vi "READ FGV.vi"(7 "Enum":T1=enum."WRITE", 8 "error in (no error)":errorcluster) -> (0 "error out":errorcluster, 3 "data":dbl[](array[numeric]) format="%.2f")   [LabVIEW 2025]
uses:
  FGV States.ctl
  CAN Write Data/Application/Common VIs/Read File Data.ctl
  <vilib>/xnet/xnet.llb/XNET Read (Signal Single-point).vi
  <vilib>/xnet/xnet.llb/XNET Create Session (Signal Input Single-point).vi
panel:
  out "DBC FUNCTIONS OUT":string[](array[string])
  out "session out 2":refnum<k21>
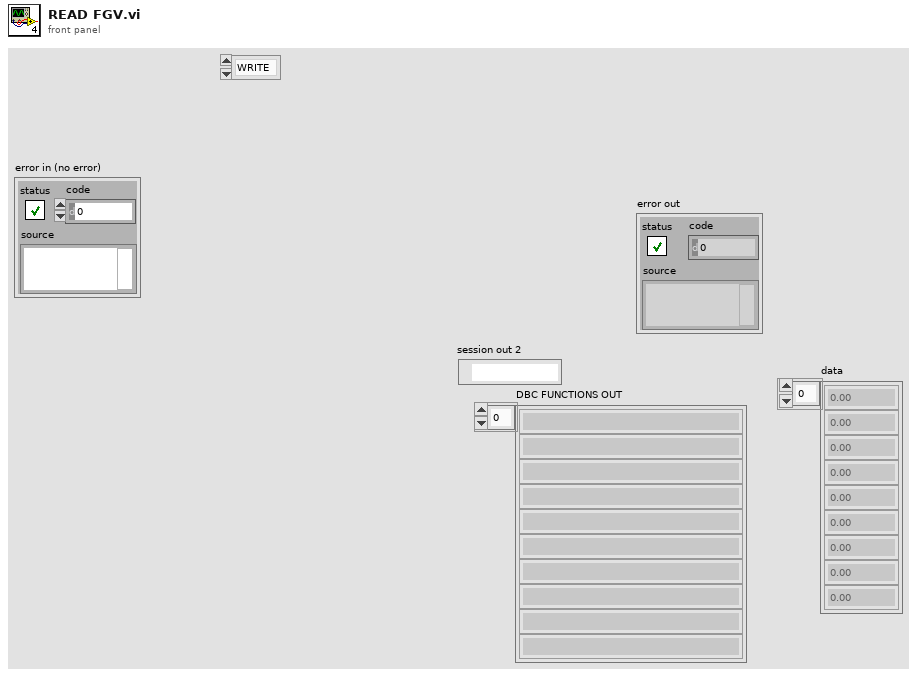
[diagram p1: front panel]
types:
  T1 = typedef "FGV States.ctl" = enum16{"OPEN", "READ", "CLOSE", "WRITE"}
  T2 = typedef "Read File Data.ctl" = enum16{"Get Data", "Set Data"}
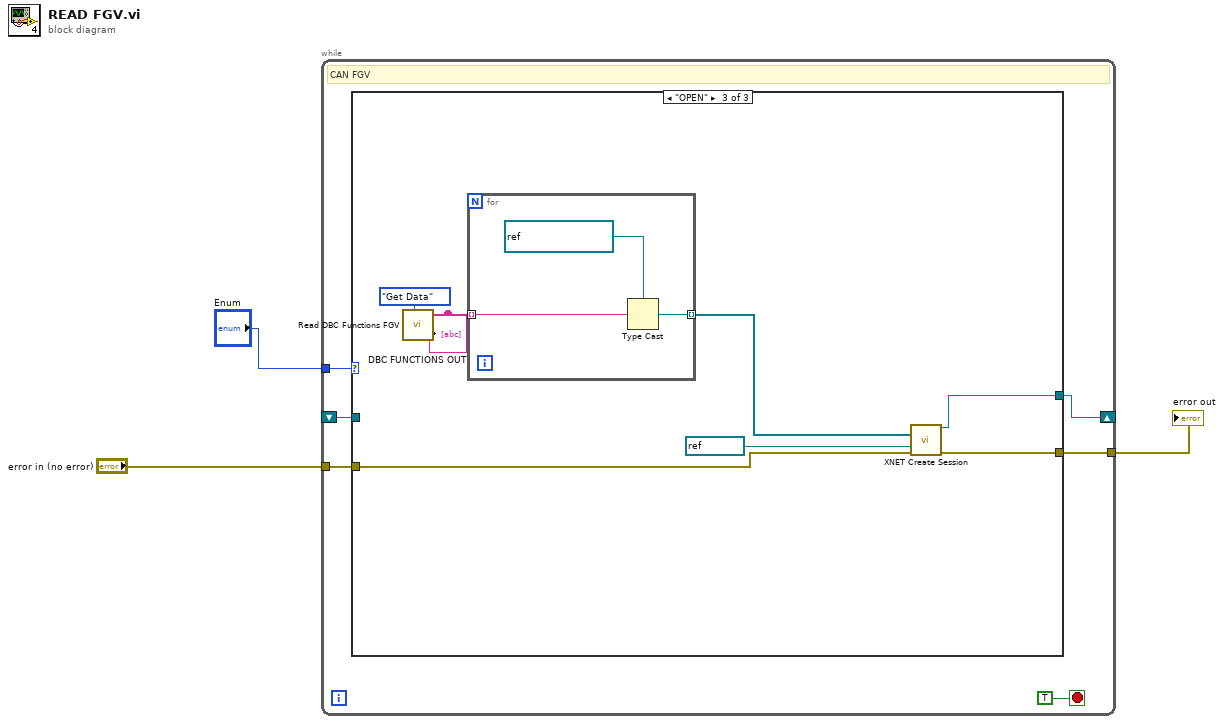
[diagram p0: block diagram]
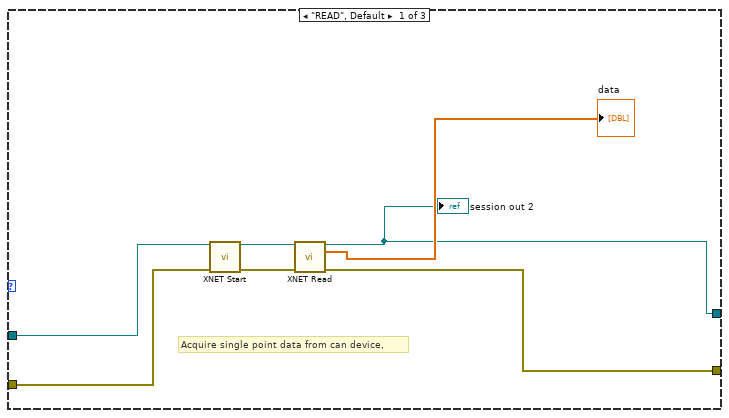
[diagram p2: hidden frame]
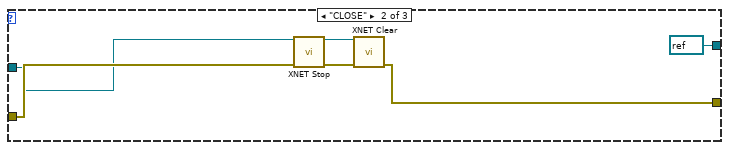
[diagram p3: hidden frame]
diagram:
  n1 = while {
    tunnel: "Enum" -> [w8]
    shift-right: [w7] -> _
    shift-left: _ -> [w6]
    tunnel: [w5] -> w1
    tunnel: "error in (no error)" -> [w4]
    stop <- TRUE stop-if-true
    # "CAN FGV"
    n2 = case shown="\"OPEN\"" w8 {
      tunnel: [w15 refnum<k21> refnum ("session out") w23] -> w7
      tunnel: w6 -> [w10 w18 _]
      tunnel: [w14 w19 w24] -> w5
      tunnel: w4 -> [w13 w20 w25]
      frame "READ", Default {
        # "Acquire single point data from can device,"
        n3 = call <vilib>:"XNET Start.vi"("session in"=w10, "error in (no error)"=w13) -> ("session out"=w11:refnum<k21>, "error out"=w12:errorcluster)  [unwired: 12 in]
        n4 = call-poly <vilib>:"XNET Read.vi"("session in"=w11, "error in (no error)"=w12) -> ("session out"=w15:refnum<k21>, "data"=→"data":dbl[], "error out"=w14:errorcluster)  [unwired: 11 in]
        "session out 2" <- w15
      }
      frame "CLOSE" {
        n5 = call <vilib>:"XNET Stop.vi"("session in"=w18, "error in (no error)"=w20) -> ("session out"=w21:refnum<k21>, "error out"=w22:errorcluster)  [unwired: 12 in]
        n6 = call <vilib>:"XNET Clear.vi"("session in"=w21, "error in (no error)"=w22) -> ("error out"=w19:errorcluster)  [unwired: 13 in]
      }
      frame "OPEN" {
        n7 = call "Read DBC Functions FGV.vi"("Enum"=Read_File_Data."Get Data") -> ("DBC FUNCTIONS OUT"=w27:string[])  [unwired: 9 in, 1 out]
        "DBC FUNCTIONS OUT" <- w27
        n8 = for {
          tunnel: w27 -> [w31] mode=indexing
          tunnel: [w30] -> w26 mode=indexing
          n9 = Type Cast(type=refnum<k21> " " ("XNET Signal"), x=w31) -> (*(type *) &x=w30:refnum<k21>)
        }
        n10 = call-poly <vilib>:"XNET Create Session.vi"("signal list"=w26, "interface"=refnum<k21> "CAN1" ("Select Interface"), "error in (no error)"=w25) -> ("session out"=w23:refnum<k21>, "error out"=w24:errorcluster)  [unwired: 11 out]
      }
    }
  }
  "error out" <- w1
